vi "Get CPU String.vi"(2 "CPU (s)":dbl) -> (7 "String":string)   [LabVIEW 2019]
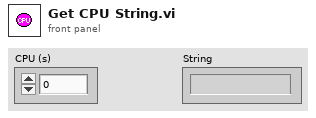
[diagram p1: front panel]
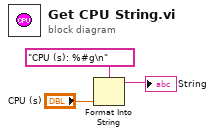
[diagram p0: block diagram]
diagram:
  n1 = Format Into String(format string="CPU (s): %#g\n", "CPU (s)") -> (resulting string=→"String":string)  [unwired: 2 in, 1 out]
